vi "Find Named Control.vi"(3 "error in":errorcluster, 4 "All Controls":refnum<vi>[](array[refnum]), 5 "Control Name":string) -> (0 "error out":errorcluster, 1 "Found":bool, 2 "Ctl Refnum":refnum<vi>)   [LabVIEW 2016]
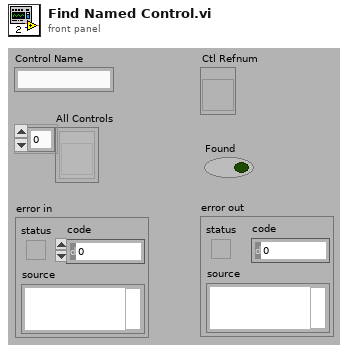
[diagram p1: front panel]
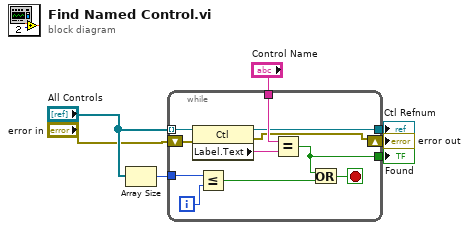
[diagram p0: block diagram]
diagram:
  n1 = Array Size(array="All Controls") -> (size(s)=w1:i32)
  n2 = while {
    tunnel: "All Controls" -> [w16] mode=indexing
    tunnel: w1 -> [w17]
    tunnel: "Control Name" -> [w14]
    tunnel: [w11] -> w4
    tunnel: [w10] -> w3
    shift-right: [w8] -> w5
    shift-left: "error in" -> [w9]
    i -> [w18]
    stop <- w13 stop-if-true
    n3 = property class="Ctl"(reference=w16, error in=w9) -> (reference out=w11:refnum<vi>, error out=w8:errorcluster, "Label.Text"=w15:string)
    n4 = Less Or Equal?(x=w17, y=w18) -> (x <= y?=w12:bool)
    n5 = Equal?(x=w14, y=w15) -> (x = y?=w10:bool)
    n6 = Or(x=w10, y=w12) -> (x .or. y?=w13:bool)
  }
  "error out" <- w5
  "Ctl Refnum" <- w4
  "Found" <- w3
